vi "AssertSourceSeparatedFromCompiledCode.vi"(8 "error in":errorcluster, 9 "folders to exclude":string[](array[string]), 10 "search path":path, 11 "TestCase in":refnum<class "TestCase.lvclass">) -> (0 "error out":errorcluster, 3 "TestCase out":refnum<class "TestCase.lvclass">)   [LabVIEW 2027, in "VeriStandTestUtilities.lvlib"]
uses:
  VeriStandTestUtilities.lvlib
  <vilib>/addons/_JKI Toolkits/VI Tester/TestCase.llb/TestCase.lvclass
  <userlib>/_OpenG.lib/file/file.llb/Append Path to Root if Relative - Scalar__ogtk.vi
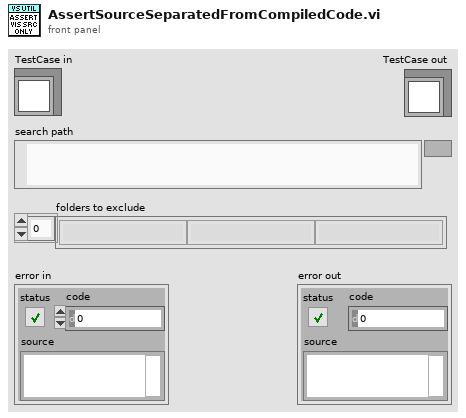
[diagram p1: front panel]
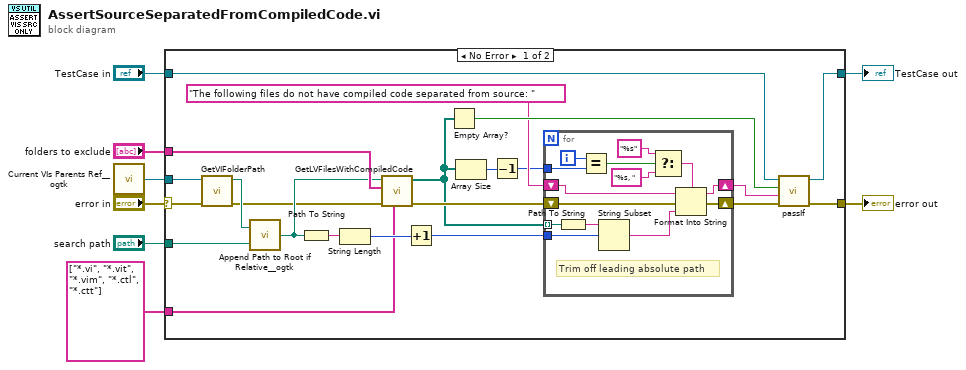
[diagram p0: block diagram]
diagram:
  n1 = call <userlib>:"Current VIs Parents Ref__ogtk.vi"() -> ("Calling VI's Reference"=w2:refnum<vi>)  [unwired: 2 in]
  n2 = case shown="No Error" "error in" {
    selector: "error in" -> [w20 w46]
    tunnel: [w28 w46] -> w8
    tunnel: "search path" -> [w18 _]
    tunnel: "TestCase in" -> [w30 w45]
    tunnel: [w29 w45] -> w4
    tunnel: "folders to exclude" -> [w13 _]
    tunnel: w2 -> [w15 _]
    tunnel: string[] ["*.vi", "*.vit", "*.vim", "*.ctl", "*.ctt"] ("patterns") -> [w9 _]
    frame No Error {
      n3 = call "GetVIFolderPath.vi"("error in (no error)"=w20, "VI Reference in"=w15) -> ("error out"=w10:errorcluster, "VI Folder Path out"=w19:path)  [unwired: 8 in]
      n4 = call-poly <userlib>:"Append Path to Root if Relative__ogtk.vi"("Absolute or Relative Path"=w18, "Root Path"=w19) -> ("Absolute or Appended Path"=w11:path)
      n5 = Path To String(path=w11) -> (string=w23:string)
      n6 = String Length(string=w23) -> (length=w22:i32)
      n7 = call "GetLVFilesWithCompiledCode.vi"("patterns"=w9, "error in"=w10, "Folders to Exclude"=w13, "Search Path"=w11) -> ("error out"=w14:errorcluster, "VIs with compiled code"=w12:path[])  [unwired: 6 in]
      n8 = Increment(x=w22) -> (x+1=w21:i32)
      n9 = Empty Array?(array=w12) -> (empty?=w27:bool)
      n10 = Array Size(array=w12) -> (size(s)=w17:i32)
      n11 = Decrement(x=w17) -> (x-1=w16:i32)
      n12 = for {
        tunnel: w12 -> [w35] mode=indexing
        shift-right: [w43] -> w25
        shift-left: "The following files do not have compiled code separated from source: " ("initial string") -> [w44]
        shift-right: [w36] -> w24
        shift-left: w14 -> [w37]
        tunnel: w21 -> [w32]
        tunnel: w16 -> [w31]
        i -> [w42]
        # "Trim off leading absolute path"
        n13 = Path To String(path=w35) -> (string=w34:string)
        n14 = Equal?(x=w42, y=w31) -> (x = y?=w39:bool)
        n15 = String Subset(string=w34, offset (0)=w32) -> (substring=w33:string)  [unwired: 1 in]
        n16 = Select(t="%s" ("format string"), s=w39, f="%s, " ("format string")) -> (s? t:f=w38:string)
        n17 = Format Into String(format string=w38, initial string=w44, error in=w37, w33) -> (resulting string=w43:string, error out=w36:errorcluster)
      }
      n18 = call-dynamic "passIf.vi"("error in (no error)"=w24, "message (\"\")"=w25, "pass"=w27, "TestCase in"=w30) -> ("error out"=w28:errorcluster, "TestCase out"=w29:refnum<class "TestCase.lvclass">)  [unwired: 6 in]
    }
    frame Error {
    }
  }
  "error out" <- w8
  "TestCase out" <- w4
